vi "test Write TagDistanceArray.vi"(8 "error in (no error)":errorcluster, 11 "TestCase in":refnum<class "AnchorTests.lvclass">) -> (0 "error out":errorcluster, 3 "TestCase out":refnum<class "AnchorTests.lvclass">)   [LabVIEW 2014, in "AnchorTests.lvclass"]
uses:
  AnchorTests.lvclass
  SPLAT/Anchor/Anchor.lvclass
  <vilib>/addons/_JKI Toolkits/VI Tester/TestCase.llb/TestCase.lvclass
  SPLAT/Tag.lvclass
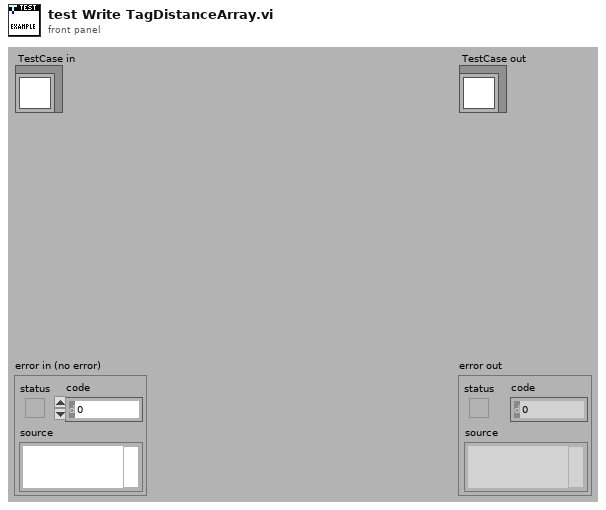
[diagram p1: front panel]
types:
  T1 = cluster{"Tag Out":refnum<class "Tag.lvclass">, "TagDistance":dbl}
  T2 = cluster{"Tag Out":refnum<class "Tag.lvclass">, "TagDistance":dbl}[]
  T3 = cluster{"Tag.lvclass":refnum<class "Tag.lvclass">, "Distance":dbl}[]
  T4 = cluster{"Tag.lvclass":refnum<class "Tag.lvclass">, "Distance":dbl}
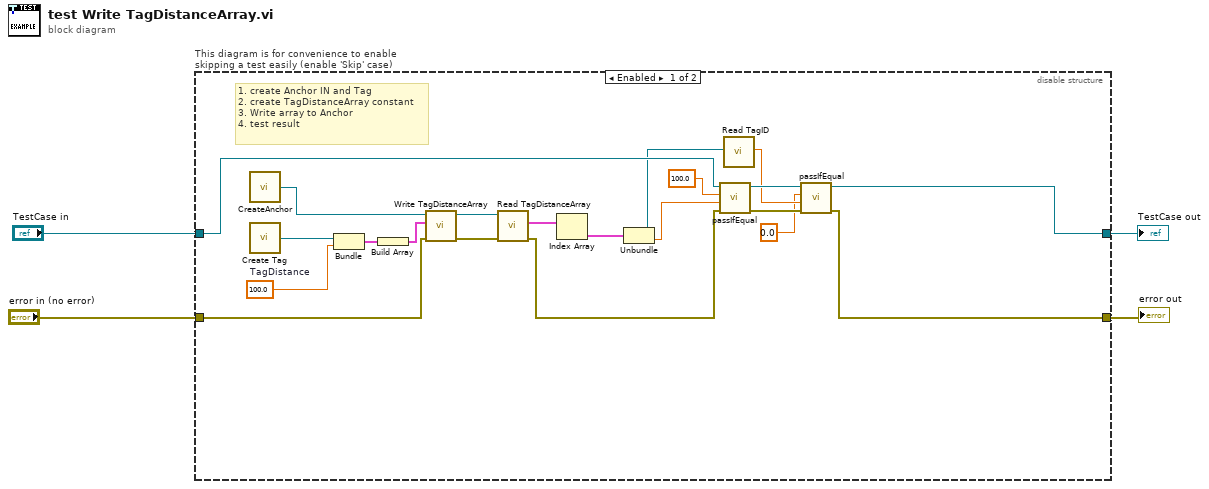
[diagram p0: block diagram]
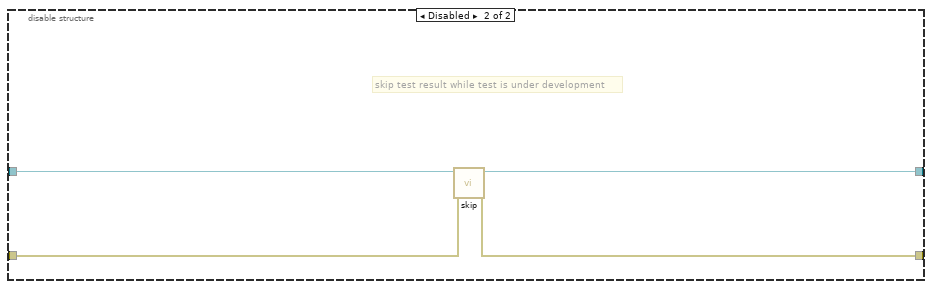
[diagram p2: hidden frame]
diagram:
  n1 = disable-structure "This diagram is for convenience to enable skipping a test easily (enable 'Skip' case)" shown="Enabled" {
    disable-tunnel: "TestCase in" -> [w19 w29]
    disable-tunnel: [w10 w27] -> w1
    disable-tunnel: [w11 w28] -> w3
    disable-tunnel: "error in (no error)" -> [w20 w26]
    frame Enabled {
      w24 = 100.0  # TagDistance
      # "1. create Anchor IN and Tag\n2. create TagDistanceArray constant\n3. Write array to Anchor\n4. test result"
      n2 = call "CreateAnchor.vi"() -> ("Anchor Out"=w21:refnum<class "Anchor.lvclass">)  [unwired: 3 in]
      n3 = call "Create Tag.vi"() -> ("Tag Out"=w25:refnum<class "Tag.lvclass">)  [unwired: 3 in]
      n4 = Bundle("Tag Out"=w25, "TagDistance"=w24) -> (w23:T1)  [unwired: 1 in]
      n5 = Build Array(w23) -> (w22:T2)
      n6 = call-dynamic "Write TagDistanceArray.vi"("error in (no error)"=w20, "TagDistanceArray"=w22, "Anchor in"=w21) -> ("error out"=w17:errorcluster, "Anchor out"=w18:refnum<class "Anchor.lvclass">)  [unwired: 7 in]
      n7 = call-dynamic "Read TagDistanceArray.vi"("error in (no error)"=w17, "Anchor in"=w18) -> ("error out"=w16:errorcluster, "TagDistanceArray"=w15:T3)  [unwired: 7 in, 1 out]
      n8 = Index Array(array=w15) -> (element=w14:T4)  [unwired: 1 in]
      n9 = Unbundle(w14) -> ("Tag.lvclass"=w8:refnum<class "Tag.lvclass">, "Distance"=w9:dbl)
      n10 = call-dynamic "passIfEqual.vi"("error in (no error)"=w16, "y"=w9, "x"=100.0, "TestCase in"=w19) -> ("error out"=w12:errorcluster, "TestCase out"=w13:refnum<class "AnchorTests.lvclass">)  [unwired: 6 in]
      n11 = call "Read TagID.vi"("Tag in"=w8) -> ("TagID"=w7:dbl)  [unwired: 16 in, 2 out]
      n12 = call-dynamic "passIfEqual.vi"("error in (no error)"=w12, "y"=w7, "x"=0.0, "TestCase in"=w13) -> ("error out"=w11:errorcluster, "TestCase out"=w10:refnum<class "AnchorTests.lvclass">)  [unwired: 6 in]
    }
    frame Disabled {
      # "skip test result while test is under development"
      n13 = call <vilib>:"skip.vi"("error in (no error)"=w26, "TestCase in"=w29) -> ("error out"=w28:errorcluster, "TestCase out"=w27:refnum<class "AnchorTests.lvclass">)  [unwired: 8 in]
    }
  }
  "error out" <- w3
  "TestCase out" <- w1
